vi "Using Queues and Callbacks.vi"() -> ()   [LabVIEW 2019]
uses:
  <userlib>/MicroPython/VIs/uPythonX/uPythonX.xctl
panel:
  in  "uPythonX":T1(xcontrol)={"Port"="Dylan pybd - ASRL117::INSTR", "All Code"="from ucollections import namedtuple\n\nMyTuple = namedtuple(\"MyTuple\", (\"id\", \"name\"))\nt1 = MyTuple(1, \"foo\")\nt2 = MyTuple(2, \"bar\")\nprint(t1.name)\nassert t2.name == t2[1]\n\nfrom ucollections import deque\nimport utime,pyb\nd = deque((), 10, 0) # 10 elements max, 1 means check overflow, 0 means FIFO\nlen(d)\n\nfor i in range(12):\n     d.append(i)\n     \nlen(d)\nfor i in range (len(d)):\n     print(d.popleft())\nlen(d)\n     \n     \nimport machine\n\n#time = machine.RTC()\n#time.init((2019,11,18,18,0,0,0))\n\ndef Ring(timerInfo):\n\n     d.append(utime.time())\n          \nsendTimer = pyb.Timer(4, freq = 0.25) # 4 sec\nsendTimer.callback(Ring)\n     \nwhile (1):\n     try:\n          print(d.popleft())\n     except:\n          utime.sleep(1)"}
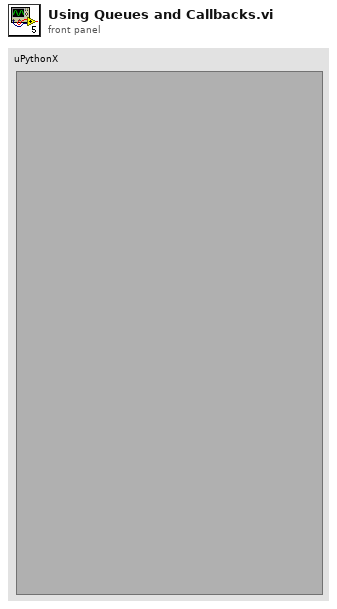
[diagram p1: front panel]
types:
  T1 = cluster{"Port":refnum<visa-resource-name>, "All Code":string}
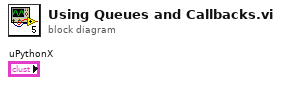
[diagram p0: block diagram]
diagram:
